vi "ident.vi"() -> ()   [LabVIEW 2011]
uses:
  <vilib>/addons/System Identification/Model Conversion.llb/SI Convert to Transfer Function Model of CDT.vi
  <vilib>/addons/Control Design/_Utility/Model Viewer.llb/Model Viewer SubVI/cd_Draw Transfer Function Equation (TF).vi
  <vilib>/addons/Control Design/_Time Response Analysis/Time Response.llb/Time Response subVI/cd_Step Response (Transfer Function).vi
  <vilib>/addons/System Identification/NI_SysID.lvlib
  <vilib>/addons/Control Design/_Time Response Analysis/NI_CD_Time Response.lvlib
  <vilib>/addons/Control Design/_Utility/NI_CD_Model Viewer.lvlib
panel:
  out "MODELO ARX TIEMPO DISCRETO":picture
  out "FUNCION DE TRANSF. TIEMPO CONT.":picture
  in  "model type":u16(ring)=1 items=["State-Space", "Transfer Function", "Zero-Pole-Gain"]
  out "RESPUESTA AL ESCALON":cluster{"time":dbl[], dbl[]}[](graph)=[{"time"=[0.0, 1.065852282082155, 2.13170456416431, 3.197556846246465, 4.26340912832862, 5.3292614104107745, 6.39511369249293, 7.460965974575085, 8.52681825665724, 9.592670538739394, 10.658522820821549, 11.724375102903705, 12.79022738498586, 13.856079667068014, 14.92193194915017, 15.987784231232325, 17.05363651331448, 18.119488795396634, 19.18534107747879, 20.251193359560943, 21.317045641643098, 22.382897923725256, 23.44875020580741, 24.514602487889565, 25.58045476997172, 26.646307052053874, 27.71215933413603, 28.778011616218183, 29.84386389830034, 30.909716180382496, 31.97556846246465, 33.041420744546805, 34.10727302662896, 35.173125308711114, 36.23897759079327, 37.30482987287542, 38.37068215495758, 39.43653443703973, 40.50238671912189, 41.56823900120404, 42.634091283286196, 43.69994356536836, 44.76579584745051, 45.83164812953267, 46.89750041161482, 47.963352693696976, 49.02920497577913, 50.095057257861285, 51.16090953994344, 52.226761822025594, 53.29261410410775, 54.3584663861899, 55.42431866827206, 56.49017095035421, 57.55602323243637, 58.62187551451852, 59.68772779660068, 60.75358007868284, 61.81943236076499, 62.88528464284715, 63.9511369249293, 65.01698920701145, 66.08284148909361, 67.14869377117576, 68.21454605325792, 69.28039833534008, 70.34625061742223, 71.41210289950439, 72.47795518158654, 73.5438074636687, 74.60965974575085, 75.67551202783301, 76.74136430991516, 77.80721659199732, 78.87306887407946, 79.93892115616163, 81.00477343824377, 82.07062572032594, 83.13647800240808, 84.20233028449024, 85.26818256657239, 86.33403484865455, 87.39988713073672, 88.46573941281886, 89.53159169490102, 90.59744397698317, 91.66329625906533, 92.72914854114748, 93.79500082322964, 94.86085310531179, 95.92670538739395], [0.0, -0.0006275688312733559, 0.026198314516787134, 0.07479645520075459, 0.13946452536577492, 0.2147322994292204, 0.2955631571514381, 0.3775035198047098, 0.45678222025917226, 0.5303636723252485, 0.5959600938662016, 0.6520089691980666, 0.6976224435526506, 0.7325154732275936, 0.7569193655381933, 0.7714868937028785, 0.7771945255935466, 0.7752465225388397, 0.7669848017796327, 0.753807564629456, 0.737098815691843, 0.7181700725950851, 0.6982148184574994, 0.6782756005144638, 0.6592231402772465, 0.6417463986468889, 0.6263522329967376, 0.6133730868214234, 0.6029810566769629, 0.5952066735025038, 0.5899608018699091, 0.5870581861809944, 0.5862413421407622, 0.5872036903675294, 0.5896110432647054, 0.5931207743070954, 0.5973982105193074, 0.6021299859268432, 0.6070342699128876, 0.6118679354224366, 0.6164308553330464, 0.6205676101894172, 0.6241669573994797, 0.6271594525745159, 0.6295136305069292, 0.631231149482446, 0.6323412817676665, 0.6328950989125576, 0.6329596566492508, 0.6326124341594909, 0.6319362295232852, 0.6310146600547709, 0.6299283653282132, 0.6287519638653295, 0.6275517730777713, 0.6263842670526775, 0.6252952186222336, 0.6243194509771436, 0.623481109653229, 0.6227943575640645, 0.6222643931980448, 0.6218886943379417, 0.6216583958098624, 0.6215597189155653, 0.6215753814545669, 0.6216859297619295, 0.6218709472177278, 0.6221101065704071, 0.6223840456177597, 0.6226750568840107, 0.6229675916152151, 0.6232485864952912, 0.6235076278708371, 0.6237369729628013, 0.6239314506100457, 0.6240882656659044, 0.6242067314296854, 0.6242879536451521, 0.6243344878568772, 0.624349989505567, 0.6243388732802837, 0.6243059951287837, 0.6242563671350824, 0.6241949123580168, 0.6241262638098949, 0.6240546091349841, 0.6239835802898936, 0.6239161856713427, 0.6238547806968734, 0.6238010718154462, 0.6237561482850784]}]
  in  "file.sim":path=path "B:/UNI/Control Digital/2013-II/Laboratorios en el MT/ARMAX/data/labview_sim_data/gate2211.sim"
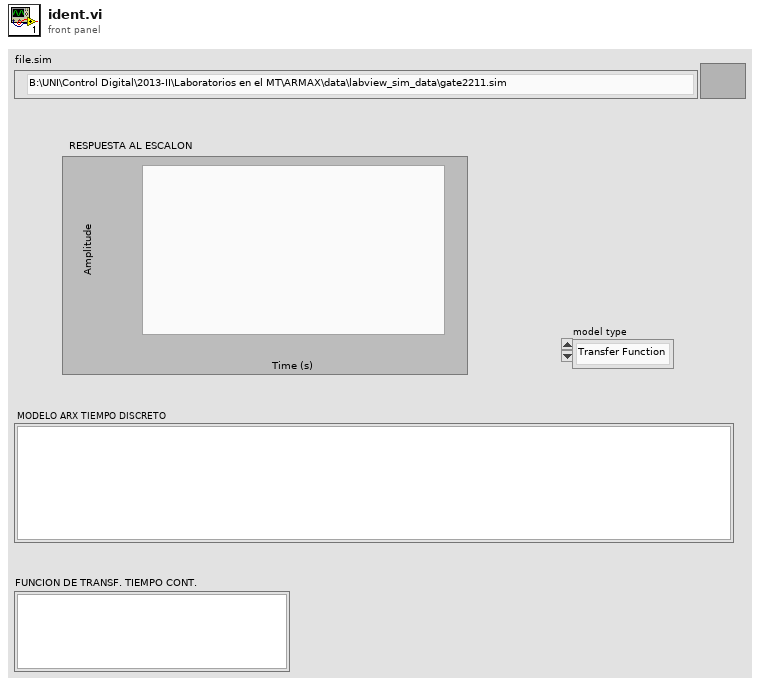
[diagram p1: front panel]
types:
  T1 = typedef "NI_SysID.lvlib/si_generic model.ctl" = cluster{"attributes":cluster{"version":string, "model type":T2, "input names":string[], "output names":string[], "notes":string}, "coefficients":cluster{"A ":dbl[][][], "B":dbl[][][], "F":dbl[][][], "C":dbl[][][], "D":dbl[][][]}, "std deviations":cluster{"A ":dbl[][][], "B":dbl[][][], "F":dbl[][][], "C":dbl[][][], "D":dbl[][][]}, "coefficients covariance":dbl[][][], "noise variance":dbl[][], "fs":dbl, "system info":cluster{"number of inputs":i32, "number of outputs":i32, "A order":i32[][], "B order":i32[][], "F order":i32[][], "C order":i32[][], "D order":i32[][], "Delays":i32[][]}, "kalman gain":dbl[][], "initial state":dbl[], "trans func":cluster{"betas":dbl[], "alphas":dbl[]}[][], "zeros-poles":cluster{"zeros":cdb[], "poles":cdb[], "gain":dbl}[][], "std of trans func":cluster{"betas":dbl[], "alphas":dbl[]}[][], "std of zeros-poles":cluster{"zeros":cdb[], "poles":cdb[], "gain":dbl}[][], "trans func (noise)":cluster{"betas":dbl[], "alphas":dbl[]}[][], "std of trans func (noise)":cluster{"betas":dbl[], "alphas":dbl[]}[][], "zeros-poles (noise)":cluster{"zeros":cdb[], "poles":cdb[], "gain":dbl}[][], "std of zeros-poles (noise)":cluster{"zeros":cdb[], "poles":cdb[], "gain":dbl}[][], "Symbolic State Space Model":cluster{"Symbolic A":string[][], "Symbolic B":string[][], "Symbolic C":string[][], "Symbolic D":string[][], "Symbolic K":string[][], "Symbolic Initial State":string[]}, "delay":dbl[][], "variables":T3, "grey trans func spec":cluster{"orders of TF model":cluster{" num order":i32, "den order":i32}, "# of zeros/poles at origin":cluster{"zeros/poles":u16, "number ":i32}, "delay initial?":bool, "gain initial?":bool}}
  T2 = typedef "NI_SysID.lvlib/SI Model Type.ctl" = u16
  T3 = typedef "NI_SysID.lvlib/si_variables.ctl" = cluster{"name":string, "initial guess":dbl, "upper limit":dbl, "lower limit":dbl, "value":dbl}[]
  T4 = typedef "NI_LinSys_Model Typedefs.lvlib/CD Transfer Function Model (MIMO).ctl" = cluster{"properties":T5, "transfer function(s)":T6[][]}
  T5 = typedef "NI_LinSys_Model Typedefs.lvlib/CD General Elements.ctl" = cluster{"Model name":string, "Input names":string[], "Output names":string[], "Input Delays":dbl[], "Output Delays":dbl[], "Sampling Time":dbl, "Notes":string}
  T6 = typedef "NI_LinSys_Model Typedefs.lvlib/CD Transfer Function Model (SISO).ctl" = cluster{"Numerator":dbl[], "Denominator":dbl[], "delay":dbl}
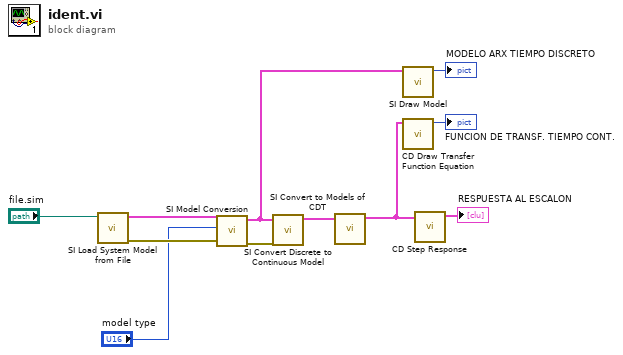
[diagram p0: block diagram]
diagram:
  n1 = call <vilib>:"SI Load System Model from File.vi"("file path"="file.sim") -> ("error out"=w9:errorcluster, "system model"=w8:T1)  [unwired: 7 in, 2 out]
  n2 = call <vilib>:"SI Model Conversion.vi"("error in (no error)"=w9, "model type"="model type", "system model in"=w8) -> ("error out"=w11:errorcluster, "system model out"=w7:T1)  [unwired: 7 in]
  n3 = call <vilib>:"SI Convert Discrete to Continuous Model.vi"("error in (no error)"=w11, "system model in"=w7) -> ("system model out"=w1:T1)  [unwired: 8 in, 1 out]
  n4 = call-poly <vilib>:"SI Convert to Models of CDT.vi"("system model"=w1) -> ("transfer function model"=w2:T4)  [unwired: 9 in, 1 out]
  n5 = call <vilib>:"SI Draw Model.vi"("system model"=w7) -> ("model"=→"MODELO ARX TIEMPO DISCRETO":picture)  [unwired: 8 in, 2 out]
  n6 = call-poly <vilib>:"CD Draw Transfer Function Equation.vi"("Transfer Function Model"=w2) -> ("Equation"=→"FUNCION DE TRANSF. TIEMPO CONT.":picture)  [unwired: 8 in, 2 out]
  n7 = call-poly <vilib>:"CD Step Response.vi"("Transfer Function Model"=w2) -> ("Step Response Graph"=→"RESPUESTA AL ESCALON":cluster{"time":dbl[], dbl[]}[])  [unwired: 8 in, 2 out]
